vi "VariantToString.vi"(11 "Variant":variant) -> (3 "String":string)   [LabVIEW 2021]
uses:
  <vilib>/Utility/VariantDataType/VariantType.lvlib
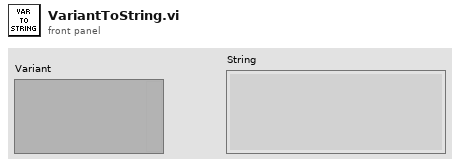
[diagram p1: front panel]
types:
  T1 = typedef "VariantType.lvlib/Type.ctl" = enum8{"Invalid Type", "Void", "I8", "I16", "I32", "I64", "U8", "U16", "U32", "U64", "Single Float", "Double Float", "Extended Float", "Single Complex", "Double Complex", "Extended Complex", "Enum U8", "Enum U16", "Enum U32", "Enum U64", "Single Float With Unit", "Double Float With Unit", "Extended Float With Unit", "Single Complex with Unit", "Double Complex with Unit", "Extended Complex with Unit", "Boolean", "String", "Path", "Picture", "Tag", "Array", "Cluster", "Variant", "LV Variant", "Waveform", "Timestamp", "Digital Waveform", "Digital Data", "ExpressData", "Refnum", "External Data", "VI", "Poly VI", "LabVIEW Class Instance", "Fixed Point"}
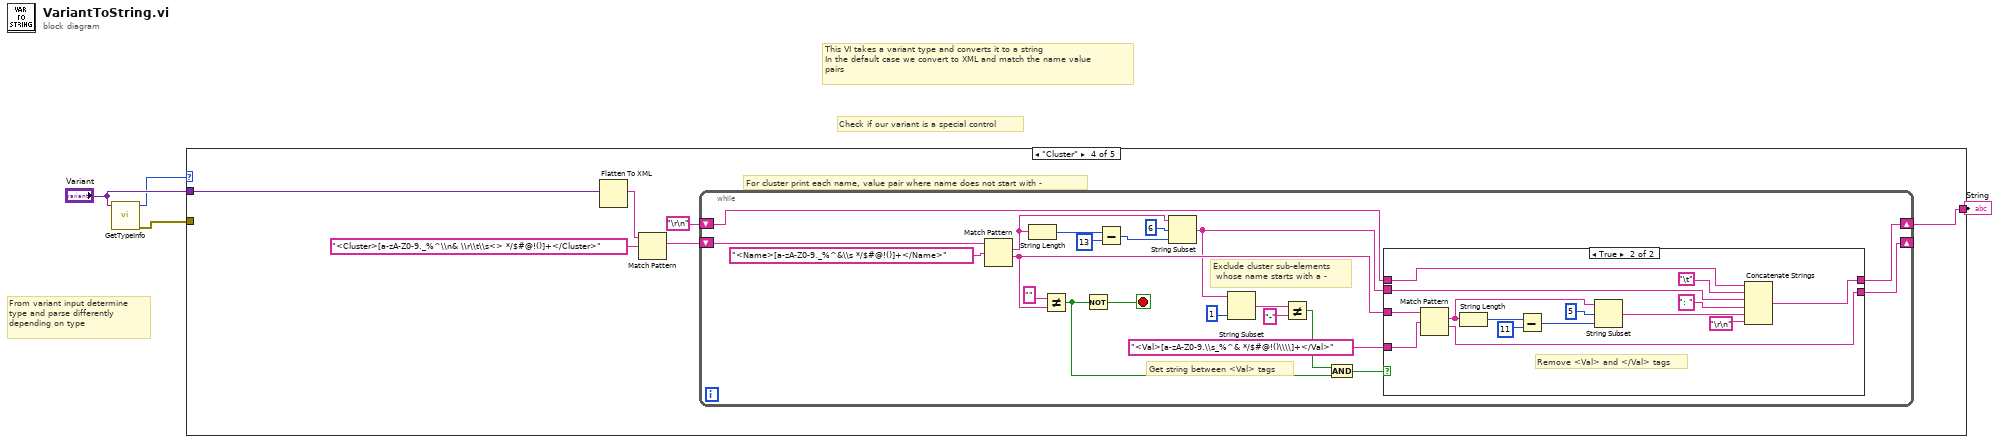
[diagram p0: block diagram]
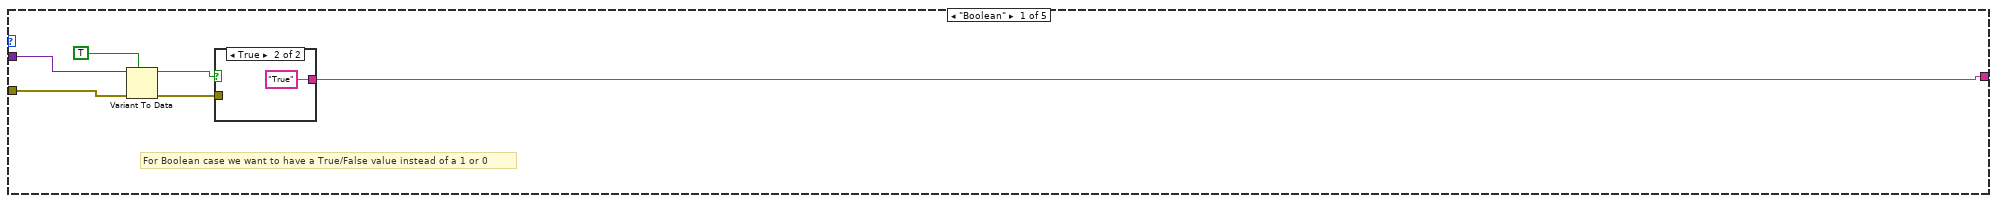
[diagram p2: hidden frame]
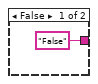
[diagram p3: hidden frame]
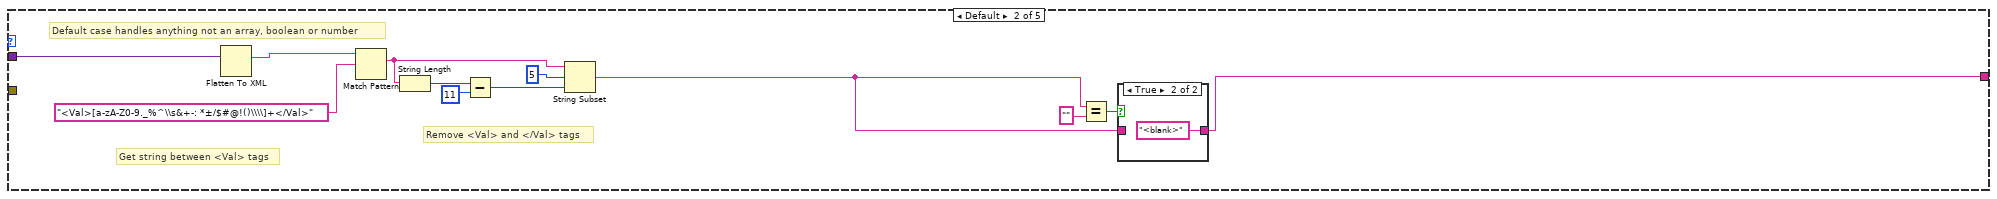
[diagram p4: hidden frame]
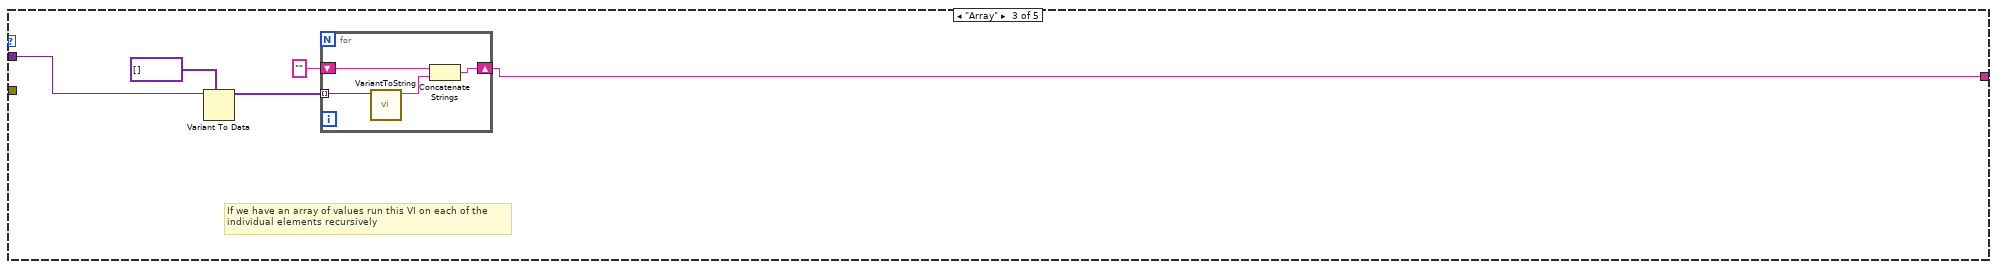
[diagram p6: hidden frame]
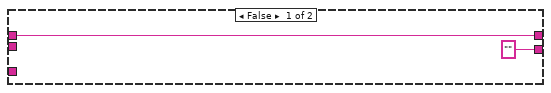
[diagram p7: hidden frame]
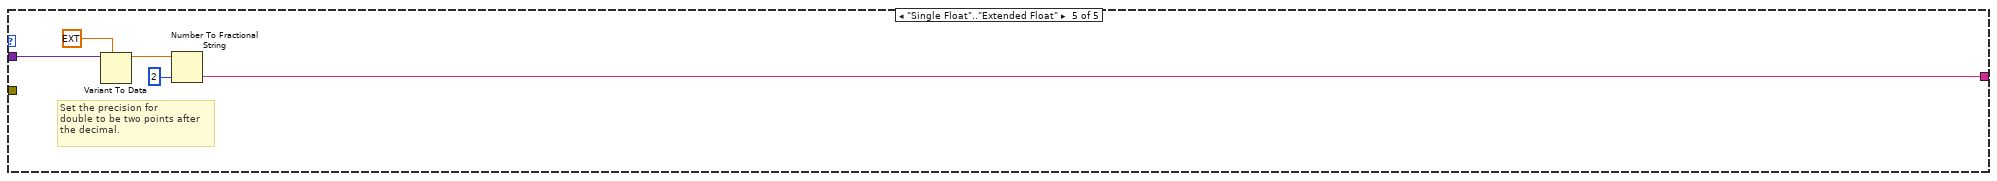
[diagram p8: hidden frame]
diagram:
  # "Check if our variant is a special control"
  # "From variant input determine\ntype and parse differently\ndepending on type"
  # "This VI takes a variant type and converts it to a string\nIn the default case we convert to XML and match the name value\npairs"
  n1 = call <vilib>:"GetTypeInfo.vi"("Variant"="Variant") -> ("error out"=w1:errorcluster, "Type Enum"=w3:T1)  [unwired: 6 in, 3 out]
  n2 = case shown="\"Cluster\"" w3 {
    tunnel: "Variant" -> [w10 w17 w31 w41 w84]
    tunnel: [w7 w13 w28 w37 w81] -> w2
    tunnel: w1 -> [w6 _ _ _ _]
    frame "Boolean" {
      # "For Boolean case we want to have a True/False value instead of a 1 or 0"
      n3 = Variant To Data(error in=w6, type=TRUE, Variant=w10) -> (data=w8:bool, error out=w5:errorcluster)
      n4 = case shown="True" w8 {
        tunnel: ["False" "True"] -> w7
        tunnel: w5 -> [_ _]
        frame False {
        }
        frame True {
        }
      }
    }
    frame Default {
      # "Default case handles anything not an array, boolean or number"
      # "Get string between <Val> tags"
      # "Remove <Val> and </Val> tags"
      n5 = Flatten To XML(6:w17) -> (2:w24:string)
      n6 = Match Pattern(string=w24, regular expression="<Val>[a-zA-Z0-9._%^\\s&+-: *±/$#@!()\\\\]+</Val>") -> (match substring=w21:string)  [unwired: 1 in, 3 out]
      n7 = String Length(string=w21) -> (length=w20:i32)
      n8 = Subtract(x=w20, y=11) -> (x-y=w18:i32)
      n9 = String Subset(string=w21, offset (0)=5, length (rest)=w18) -> (substring=w15:string)
      n10 = Equal?(x=w15, y="") -> (x = y?=w14:bool)
      n11 = case shown="True" w14 {
        tunnel: w15 -> [w25 _]
        tunnel: [w25 "<blank>" ("xml string")] -> w13
        frame False {
        }
        frame True {
        }
      }
    }
    frame "Array" {
      # "If we have an array of values run this VI on each of the\nindividual elements recursively"
      n12 = Variant To Data(type=variant[] [], Variant=w31) -> (data=w29:variant[])  [unwired: 1 in, 1 out]
      n13 = for {
        tunnel: w29 -> [w35] mode=indexing
        shift-right: [w34] -> w28
        shift-left: "" -> [w33]
        n14 = call <vilib>:"VariantToString.vi"("Variant"=w35) -> ("String"=w32:string)  [unwired: 10 in]
        n15 = Concatenate Strings(w33, w32) -> (w34:string)
      }
    }
    frame "Cluster" {
      # "For cluster print each name, value pair where name does not start with -"
      n16 = Flatten To XML(6:w41) -> (2:w40:string)
      n17 = Match Pattern(string=w40, regular expression="<Cluster>[a-zA-Z0-9._%^\\n& \\r\\t\\s<> */$#@!()]+</Cluster>") -> (match substring=w38:string)  [unwired: 1 in, 3 out]
      n18 = while {
        shift-right: [w58] -> _
        shift-left: w38 -> [w61]
        shift-right: [w59] -> w37
        shift-left: "\r\n" -> [w57]
        stop <- w54 stop-if-true
        # "Get string between <Val> tags"
        # "Exclude cluster sub-elements\n whose name starts with a -"
        n19 = Match Pattern(string=w61, regular expression="<Name>[a-zA-Z0-9._%^&\\s */$#@!()]+</Name>") -> (match substring=w49:string, after substring=w56:string)  [unwired: 1 in, 2 out]
        n20 = String Length(string=w49) -> (length=w52:i32)
        n21 = Not Equal?(x="", y=w56) -> (x != y?=w48:bool)
        n22 = Not(x=w48) -> (.not. x?=w54:bool)
        n23 = Subtract(x=w52, y=13) -> (x-y=w50:i32)
        n24 = String Subset(string=w49, offset (0)=6, length (rest)=w50) -> (substring=w47:string)
        n25 = String Subset(string=w47, length (rest)=1 ("length (rest)")) -> (substring=w45:string)  [unwired: 1 in]
        n26 = Not Equal?(x=w45, y="-") -> (x != y?=w43:bool)
        n27 = And(x=w43, y=w48) -> (x .and. y?=w42:bool)
        n28 = case shown="True" w42 {
          tunnel: "<Val>[a-zA-Z0-9.\\s_%^& */$#@!()\\\\]+</Val>" ("regular expression") -> [_ w79]
          tunnel: [w63 w77] -> w59
          tunnel: ["" ("xml string") w76] -> w58
          tunnel: w57 -> [w63 w66]
          tunnel: w56 -> [_ w75]
          tunnel: w47 -> [_ w74]
          frame False {
          }
          frame True {
            # "Remove <Val> and </Val> tags"
            n29 = Match Pattern(string=w75, regular expression=w79) -> (match substring=w68:string, after substring=w76:string)  [unwired: 1 in, 2 out]
            n30 = String Length(string=w68) -> (length=w72:i32)
            n31 = Subtract(x=w72, y=11) -> (x-y=w70:i32)
            n32 = String Subset(string=w68, offset (0)=5, length (rest)=w70) -> (substring=w69:string)
            n33 = Concatenate Strings(w66, "\t", w74, ": " ("string"), w69, "\r\n") -> (w77:string)
          }
        }
      }
    }
    frame "Single Float".."Extended Float" {
      # "Set the precision for\ndouble to be two points after\nthe decimal."
      n34 = Variant To Data(type=ext 0.0, Variant=w84) -> (data=w82:ext)  [unwired: 1 in, 1 out]
      n35 = Number To Fractional String(number=w82, precision (6)=i16 2) -> (F-format string=w81:string)  [unwired: 2 in]
    }
  }
  "String" <- w2
